vi "绘制选择框.vi"(8 "error in (no error)":errorcluster caption="错误输入（无错误）", 11 "程序 输入":refnum<class "程序.lvclass">) -> (0 "error out":errorcluster caption="错误输出", 3 "程序 输出":refnum<class "程序.lvclass">)   [LabVIEW 2020, in "程序.lvclass"]
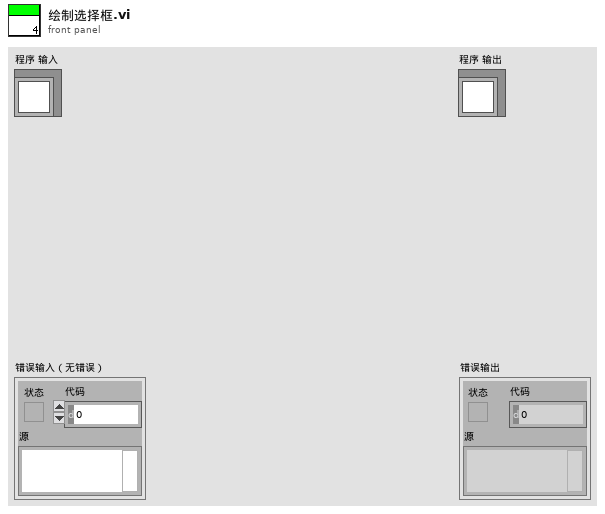
[diagram p1: front panel]
types:
  T1 = cluster{"Width":i16, "Style":enum32{"Solid", "Dash", "Dot", "DashDot", "DashDotDot"}}
  T2 = typedef "LVPositionTypeDef.ctl" = cluster{"Left":i32, "Top":i32}
  T3 = typedef "LVBoundsTypeDef.ctl" = cluster{"Width":u32, "Height":u32}
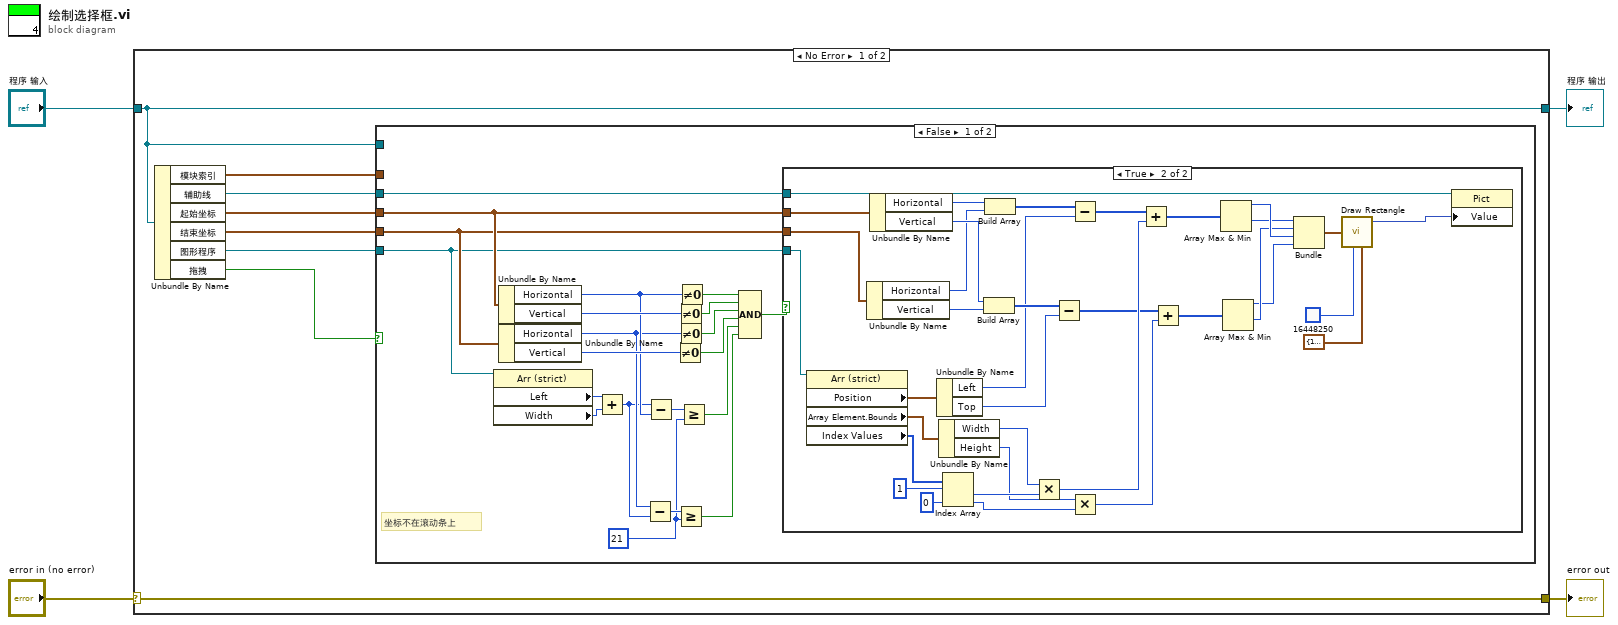
[diagram p0: block diagram]
diagram:
  n1 = case shown="No Error" "error in (no error)" {
    selector: "error in (no error)" -> [w12 w70]
    tunnel: [w12 w70] -> w3
    tunnel: [w6 w69] -> w1
    tunnel: "程序 输入" -> [w6 w69]
    frame No Error {
      n2 = Unbundle By Name(w6) -> ("模块索引"=w7:cluster{"列":u32, "行":u32}, "辅助线"=w11:refnum<vi>, "起始坐标"=w10:cluster{"Horizontal":i32, "Vertical":i32}, "结束坐标"=w9:cluster{"Horizontal":i32, "Vertical":i32}, "图形程序"=w8:refnum<vi>, "拖拽"=w5:bool)
      n3 = case shown="False" w5 {
        tunnel: w11 -> [w33 _]
        tunnel: w10 -> [w32 _]
        tunnel: w9 -> [w31 _]
        tunnel: w8 -> [w20 _]
        tunnel: w7 -> [_ _]
        tunnel: w6 -> [_ _]
        frame False {
          w13 = u32 21 ("y")
          # "坐标不在滚动条上"
          n4 = property class="Arr (strict)"(reference=w20) -> ("Left"=w21:i32, "Width"=w22:u32)  [unwired: 1 in, 2 out]
          n5 = Unbundle By Name(w32) -> ("Horizontal"=w19:i32, "Vertical"=w30:i32)
          n6 = Unbundle By Name(w31) -> ("Horizontal"=w17:i32, "Vertical"=w29:i32)
          n7 = Add(x=w21, y=w22) -> (x+y=w16:u32)
          n8 = Subtract(x=w17, y=w16) -> (x-y=w18:u32)
          n9 = Subtract(x=w16, y=w19) -> (x-y=w23:u32)
          n10 = Not Equal To 0?(x=w29) -> (x != 0?=w25:bool)
          n11 = Not Equal To 0?(x=w30) -> (x != 0?=w27:bool)
          n12 = Not Equal To 0?(x=w17) -> (x != 0?=w26:bool)
          n13 = Greater Or Equal?(x=w18, y=w13) -> (x >= y?=w14:bool)
          n14 = Not Equal To 0?(x=w19) -> (x != 0?=w28:bool)
          n15 = Greater Or Equal?(x=w23, y=w13) -> (x >= y?=w15:bool)
          n16 = Compound Arithmetic op=AND ("复合运算")(w28, w27, w26, w25, w15, w14) -> (w24:bool)
          n17 = case shown="True" w24 {
            tunnel: w33 -> [_ w51]
            tunnel: w32 -> [_ w54]
            tunnel: w31 -> [_ w53]
            tunnel: w20 -> [_ w50]
            frame False {
            }
            frame True {
              n18 = property class="Arr (strict)"(reference=w50) -> ("Position"=w57:T2, "Array Element.Bounds"=w49:T3, "Index Values"=w48:u32[])  [unwired: 1 in, 2 out]
              n19 = Unbundle By Name(w53) -> ("Horizontal"=w61:i32, "Vertical"=w63:i32)
              n20 = Unbundle By Name(w54) -> ("Horizontal"=w60:i32, "Vertical"=w62:i32)
              n21 = Unbundle By Name(w57) -> ("Left"=w41:i32, "Top"=w40:i32)
              n22 = Unbundle By Name(w49) -> ("Width"=w45:u32, "Height"=w43:u32)
              n23 = Index Array(array=w48, index #1=1 ("索引"), index #2=0 ("索引")) -> (element #1=w44:u32, element #2=w42:u32)
              n24 = Build Array(w62, w63) -> (w55:i32[])
              n25 = Build Array(w60, w61) -> (w56:i32[])
              n26 = Multiply(x=w45, y=w44) -> (x*y=w38:u32)
              n27 = Subtract(x=w55, y=w40) -> (x-y=w36:i32[])
              n28 = Subtract(x=w56, y=w41) -> (x-y=w39:i32[])
              n29 = Multiply(x=w43, y=w42) -> (x*y=w34:u32)
              n30 = Add(x=w39, y=w38) -> (x+y=w37:u32[])
              n31 = Add(x=w36, y=w34) -> (x+y=w35:u32[])
              n32 = Array Max & Min(array=w37) -> (max value=w66:u32, min value=w64:u32)  [unwired: 2 out]
              n33 = Array Max & Min(array=w35) -> (max value=w58:u32, min value=w65:u32)  [unwired: 2 out]
              n34 = Bundle(w64, w65, w66, w58) -> (w59:cluster{u32, u32, u32, u32})  [unwired: 1 in]
              n35 = call <vilib>:"Draw Rectangle.vi"("rect"=w59, "color(black)"=u32 16448250, "pen"=T1 {"Width"=1, "Style"=enum."Dot"}) -> ("new picture"=w68:picture)  [unwired: 6 in]
              n36 = property class="Pict"(reference=w51, "Value"=w68) -> ()  [unwired: 1 in, 2 out]
            }
          }
        }
        frame True {
        }
      }
    }
    frame Error {
    }
  }
  "error out" <- w3
  "程序 输出" <- w1
